vi "Initialise cRIO.vi"(3 "State Ring":u16(ring) items=["Init VI", "Init Event Handlers", "Booting sequence", "Operational", "Emergency shutting down", "Shuting down", "Closing VI"], 7 "error in":errorcluster) -> (13 "Shutdown Notifier":refnum<notifier>, 15 "Emergency Turn Off Notifier":refnum<notifier>, 19 "Update Motors Notifier":refnum<notifier>, 20 "Log File Cluster":T1, 21 "CANOpen Session":refnum<k20>, 22 "CAN Session":T3, 26 "Error Queue":refnum<queue>, 27 "error out":errorcluster)   [LabVIEW 2016]
uses:
  Program Files (x86)/National Instruments/LabVIEW 2016/examples/robotics/EPOS2 CANOpen Driver/Low Level VIs/Typedefs/CAN Refnum.ctl
  Program Files (x86)/National Instruments/LabVIEW 2016/examples/robotics/EPOS2 CANOpen Driver/Low Level VIs/Typedefs/CAN Session Pointer.ctl
  Program Files (x86)/National Instruments/LabVIEW 2016/examples/robotics/EPOS2 CANOpen Driver/Low Level VIs/Typedefs/CAN Communication References.ctl
  Program Files (x86)/National Instruments/LabVIEW 2016/examples/robotics/EPOS2 CANOpen Driver/Low Level VIs/Typedefs/kill process notifier array.ctl
  Program Files (x86)/National Instruments/LabVIEW 2016/examples/robotics/EPOS2 CANOpen Driver/Low Level VIs/Typedefs/Write Queue.ctl
  Program Files (x86)/National Instruments/LabVIEW 2016/examples/robotics/EPOS2 CANOpen Driver/Low Level VIs/Typedefs/FPGA CAN Frame Cluster.ctl
  Tests/Log File Cluster.ctl
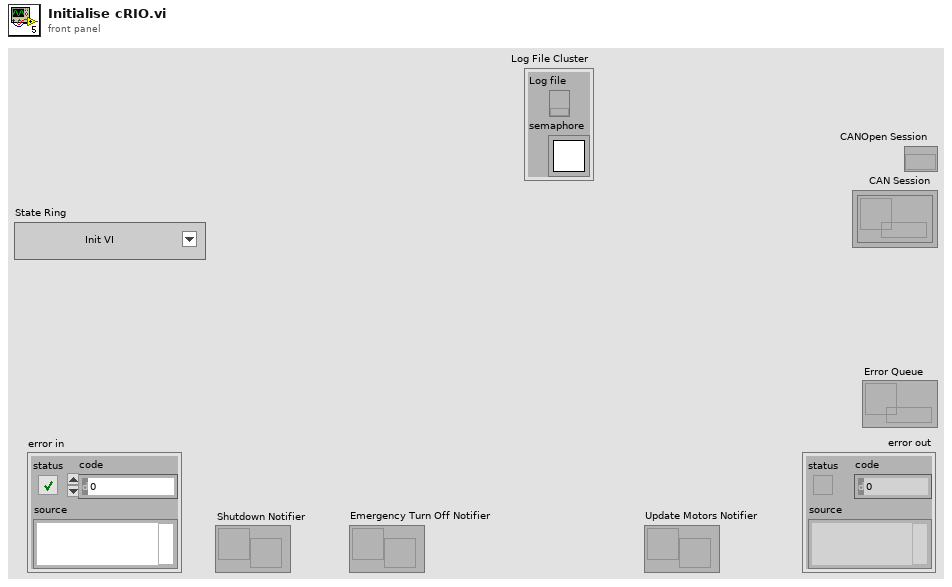
[diagram p1: front panel]
types:
  T1 = typedef "Log File Cluster.ctl" = cluster{"Log file":refnum<k34>, "semaphore":T2}
  T2 = typedef "Semaphore RefNum" = refnum<k1>
  T3 = typedef "CAN Refnum.ctl" = refnum<k1>
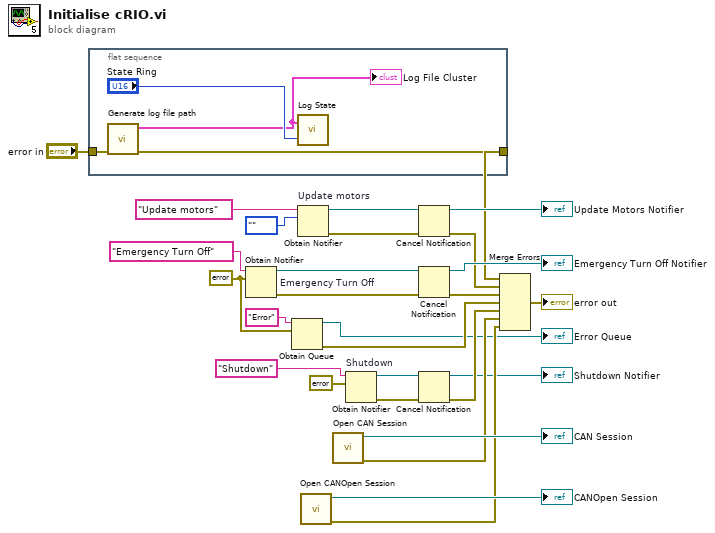
[diagram p0: block diagram]
diagram:
  w3 = errorcluster {"status"=FALSE, "code"=0, "source"=""} ("error constant")
  n1 = flat-sequence {
    tunnel: "error in" -> [w32]
    tunnel: [w31] -> w18
    frame #0 {
      n2 = call "Generate log file path.vi"("error in"=w32) -> ("error out"=w31:errorcluster, "Log File Cluster"=w29:T1)  [unwired: 9 in]
      "Log File Cluster" <- w29
      n3 = call "Log State.vi"("State Ring"="State Ring", "Log File Cluster"=w29) -> ()  [unwired: 1 in]
    }
  }
  n4 = Obtain Notifier "Emergency Turn Off"(name (unnamed)="Emergency Turn Off", notification data type=w3) -> (notifier out=w27:refnum<notifier>, error out=w25:errorcluster)  [unwired: 2 in, 1 out]
  n5 = Obtain Queue(name (unnamed)="Error", element data type=w3) -> (queue out=→"Error Queue":refnum<queue>, error out=w2:errorcluster)  [unwired: 3 in, 1 out]
  n6 = Obtain Notifier "Update motors"(name (unnamed)="Update motors", notification data type=enum16{""}."") -> (notifier out=w23:refnum<notifier>, error out=w24:errorcluster)  [unwired: 2 in, 1 out]
  n7 = call "Open CANOpen Session.vi"() -> ("error out"=w14:errorcluster, "interface object out"=→"CANOpen Session":refnum<k20>)  [unwired: 10 in]
  n8 = call "Open CAN Session.vi"() -> ("error out"=w15:errorcluster, "CAN Session"=→"CAN Session":T3)  [unwired: 10 in]
  n9 = Obtain Notifier "Shutdown"(name (unnamed)="Shutdown", notification data type=errorcluster {"status"=FALSE, "code"=0, "source"=""} ("error constant")) -> (notifier out=w7:refnum<notifier>, error out=w12:errorcluster)  [unwired: 2 in, 1 out]
  n10 = Cancel Notification(0:w23, 3:w24) -> (8:→"Update Motors Notifier":refnum<notifier>, 11:w17:errorcluster)  [unwired: 1 out]
  n11 = Cancel Notification(0:w27, 3:w25) -> (8:→"Emergency Turn Off Notifier":refnum<notifier>, 11:w16:errorcluster)  [unwired: 1 out]
  n12 = Cancel Notification(0:w7, 3:w12) -> (8:→"Shutdown Notifier":refnum<notifier>, 11:w6:errorcluster)  [unwired: 1 out]
  n13 = Merge Errors(w18, w17, w16, w2, w6, w15, w14) -> (→"error out":errorcluster)
